vi "例6.1 利用文本文件IO保存数据.vi"() -> ()   [LabVIEW 2017]
panel:
  in  "文件路径（使用对话框）":path=path "D:/1.TXT"
  in  "写入的点数":dbl=5.0
  out "波形图表":i32(graph)
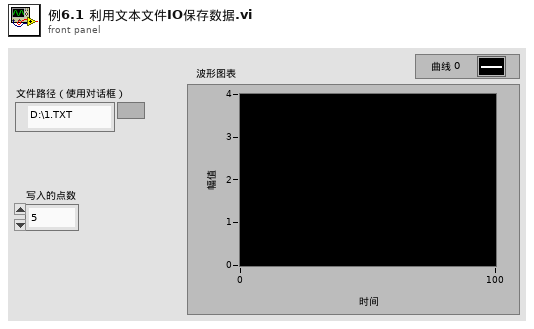
[diagram p1: front panel]
types:
  T1 = enum16{"open", "replace", "create", "open or create", "replace or create", "replace or create with confirmation"}
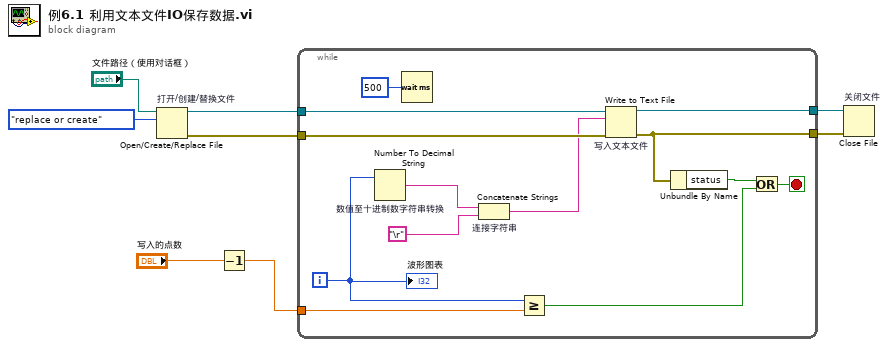
[diagram p0: block diagram]
diagram:
  n1 = Open/Create/Replace File "打开/创建/替换文件"(file path (use dialog)="文件路径（使用对话框）", operation (0:open)=T1."replace or create" ("操作(0:open)")) -> (refnum out=w8:refnum<file>, error out=w6:errorcluster)  [unwired: 4 in, 1 out]
  n2 = Decrement(x="写入的点数") -> (x-1=w3:dbl)
  n3 = while {
    tunnel: w8 -> [w21]
    tunnel: [w20] -> w7
    tunnel: w6 -> [w19]
    tunnel: [w17] -> w5
    tunnel: w3 -> [w18]
    i -> [w9]
    stop <- w14 stop-if-true
    n4 = Number To Decimal String "数值至十进制数字符串转换"(number=w9) -> (decimal integer string=w12:string)  [unwired: 1 in]
    n5 = Wait (ms)(milliseconds to wait=u32 500 ("等待时间（毫秒）")) -> ()  [unwired: 1 out]
    n6 = Concatenate Strings "连接字符串"(w12, "\r") -> (w10:string)
    n7 = Greater Or Equal?(x=w9, y=w18) -> (x >= y?=w15:bool)
    n8 = Write to Text File "写入文本文件"(file (use dialog)=w21, text=w10, error in=w19) -> (refnum out=w20:refnum<file>, error out=w17:errorcluster)  [unwired: 1 in, 1 out]
    n9 = Unbundle By Name(w17) -> ("status"=w16:bool)
    n10 = Or(x=w16, y=w15) -> (x .or. y?=w14:bool)
    "波形图表" <- w9
  }
  n11 = Close File "关闭文件"(refnum=w7, error in=w5) -> ()  [unwired: 2 out]
